vi "Interruptible Timer.vi"(8 "error in (no error)":errorcluster, 10 "Update UI?":bool, 11 "Wait (s)":i32) -> (0 "error out":errorcluster, 2 "Time Elapsed":u32, 3 "Aborted?":bool)   [LabVIEW 2015]
uses:
  User Interface/UI Handler/UI Handler.lvclass
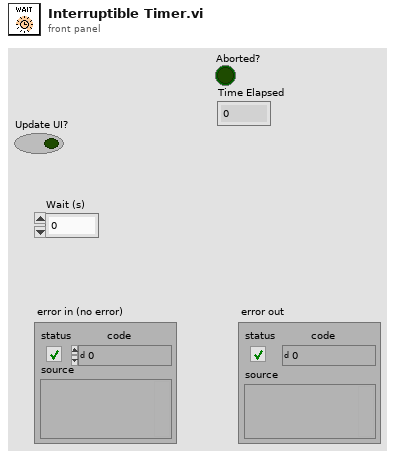
[diagram p1: front panel]
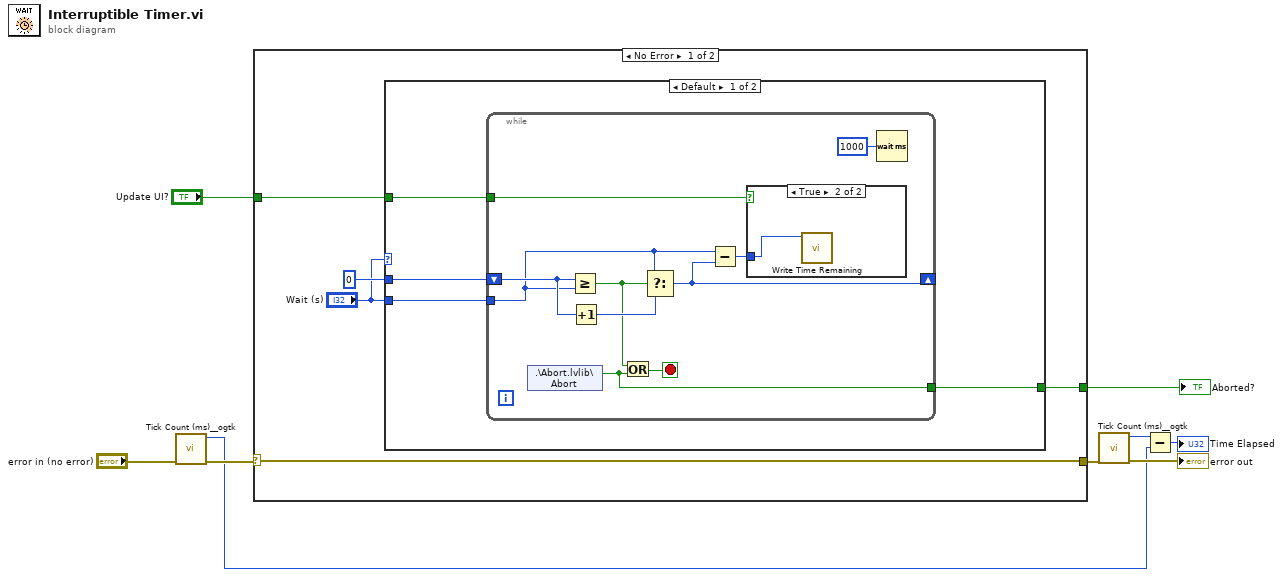
[diagram p0: block diagram]
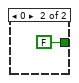
[diagram p3: hidden frame]
diagram:
  n1 = call <userlib>:"Tick Count (ms)__ogtk.vi"("error in (no error)"="error in (no error)") -> ("error out"=w7:errorcluster, "millisecond timer value"=w3:u32)  [unwired: 9 in]
  n2 = case shown="No Error" w7 {
    selector: w7 -> [w13 w31]
    tunnel: [w13 w31] -> w6
    tunnel: [w12 _] -> w9
    tunnel: "Update UI?" -> [w11 _]
    frame No Error {
      n3 = case shown="Default" "Wait (s)" {
        tunnel: "Wait (s)" -> [w18 _]
        tunnel: 0 -> [w17 _]
        tunnel: [w16 FALSE ("Boolean")] -> w12
        tunnel: w11 -> [w15 _]
        frame Default {
          n4 = while {
            tunnel: w18 -> [w22]
            shift-right: [w23] -> _
            shift-left: w17 -> [w28]
            tunnel: [w24] -> w16
            tunnel: w15 -> [w20]
            stop <- w26 stop-if-true
            n5 = shared-variable ".\\Abort.lvlib\\Abort"() -> (w24:bool)  [unwired: 1 in, 1 out]
            n6 = Greater Or Equal?(x=w28, y=w22) -> (x >= y?=w25:bool)
            n7 = Increment(x=w28) -> (x+1=w27:i32)
            n8 = Or(x=w25, y=w24) -> (x .or. y?=w26:bool)
            n9 = Select(t=w22, s=w25, f=w27) -> (s? t:f=w23:i32)
            n10 = Subtract(x=w22, y=w23) -> (x-y=w21:i32)
            n11 = case shown="True" w20 {
              tunnel: w21 -> [_ w29]
              frame False {
              }
              frame True {
                n12 = call "Write Time Remaining.vi"("Value"=w29) -> ()  [unwired: 10 in, 1 out]
              }
            }
            n13 = Wait (ms)(milliseconds to wait=u32 1000) -> ()  [unwired: 1 out]
          }
        }
        frame 0 {
        }
      }
    }
    frame Error {
    }
  }
  "Aborted?" <- w9
  n14 = call <userlib>:"Tick Count (ms)__ogtk.vi"("error in (no error)"=w6) -> ("error out"=→"error out":errorcluster, "millisecond timer value"=w4:u32)  [unwired: 9 in]
  n15 = Subtract(x=w4, y=w3) -> (x-y=→"Time Elapsed":u32)
